vi "Beta 2.1.vi"() -> ()   [LabVIEW 2011]
uses:
  <vilib>/vision/NI_Vision_Development_Module.lvlib
panel:
  in  "OK Button":bool
  in  "Look for":enum16{"Bright Objects", "Dark Objects"}(ring)
  in  "Method":T1(ring)=enum."Inter-class Variance"
  out "Binary":T2(plugin-control)
  out "Threshold Range":cluster{"Lower value":sgl, "Upper value":sgl}={"Lower value"=128.0, "Upper value"=255.0} {"Upper value" format="%.2f"; "Lower value" format="%.2f"}
  in  "Stop":bool
  in  "Browse":bool
  out "XY Graph":cluster{dbl[], dbl[]}(graph)
  out "Original Image":T2(plugin-control)
  out "Path to Image":path
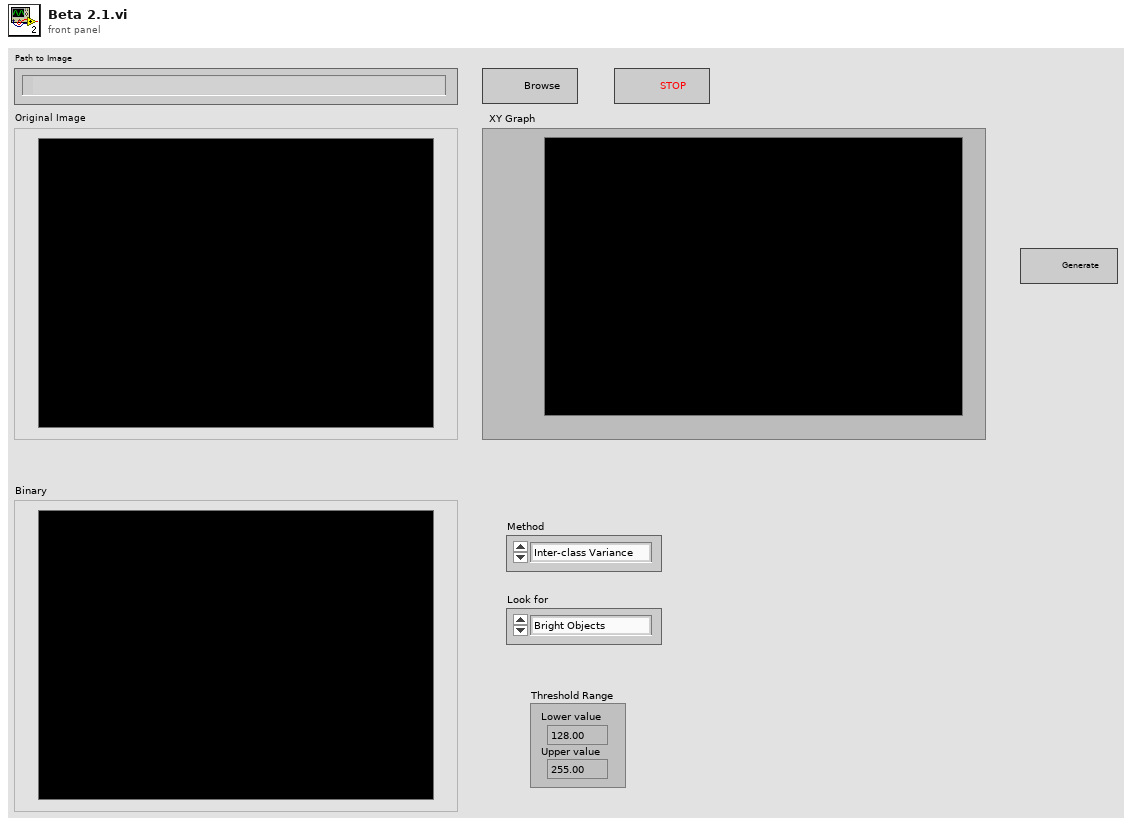
[diagram p1: front panel]
types:
  T1 = enum16{"Clustering", "Entropy", "Metric", "Moments", "Inter-class Variance"}
  T2 = typedef "IMAQ Image.ctl" = refnum<image>
  T3 = typedef "Image Type" = u32
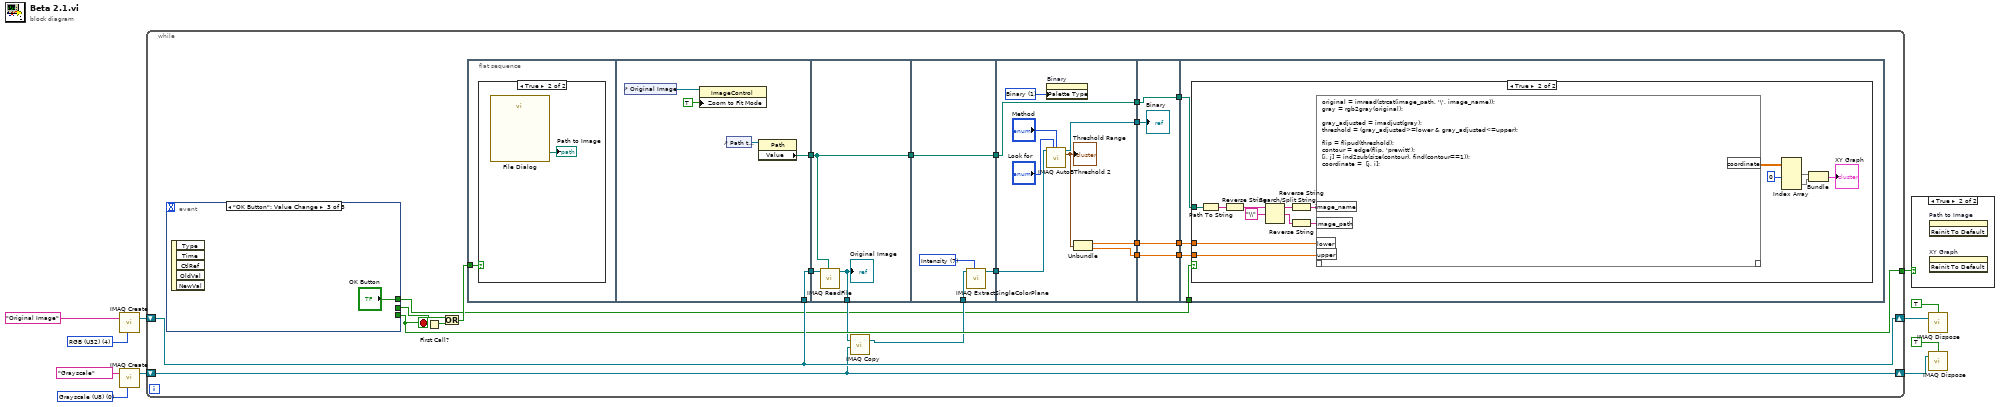
[diagram p0: block diagram]
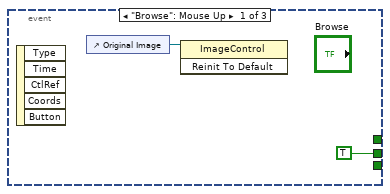
[diagram p3: hidden frame]
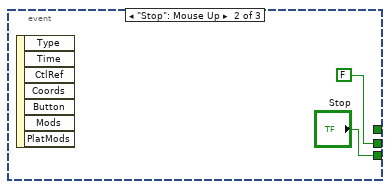
[diagram p4: hidden frame]
diagram:
  w5 = T3 0 items=["Grayscale (U8)", "Grayscale (I16)", "Grayscale (SGL)", "Complex (CSG)", "RGB (U32)", "HSL (U32)", "RGB (U64)", "Grayscale (U16)"] ("Image Type")
  w10 = T3 4 items=["Grayscale (U8)", "Grayscale (I16)", "Grayscale (SGL)", "Complex (CSG)", "RGB (U32)", "HSL (U32)", "RGB (U64)", "Grayscale (U16)"] ("Image Type")
  n1 = call "IMAQ Create"("Image Name"="Original Image", "Image Type"=w10) -> ("New Image"=w9:T2)  [unwired: 3 in, 1 out]
  n2 = call "IMAQ Create"("Image Name"="Grayscale", "Image Type"=w5) -> ("New Image"=w4:T2)  [unwired: 3 in, 1 out]
  n3 = while {
    shift-right: [w27] -> w8
    shift-left: w9 -> [w27]
    tunnel: [w26] -> w7
    shift-right: [w17] -> w2
    shift-left: w4 -> [w17]
    stop <- w26 stop-if-true
    n4 = event shown="[2] \"OK Button\": Value Change" {
      selector: _ -> [_ _ _]
      dyn-events: _ -> [_ _ _]
      timeout: _ -> [_ _ _]
      tunnel: [TRUE FALSE _] -> w31
      tunnel: [_ "Stop" _] -> w26
      tunnel: [_ _ "OK Button"] -> w16
      event "Browse": Mouse Up {
        n5 = event-data() -> ()  [unwired: 1 in, 5 out]
        n6 = control-ref of="Original Image"() -> (w34:refnum<vi>)
        n7 = invoke class="ImageControl" method="Reinit To Default"(reference=w34) -> ()  [unwired: 2 in, 3 out]
      }
      event "Stop": Mouse Up {
        n8 = event-data() -> ()  [unwired: 1 in, 7 out]
      }
      event "OK Button": Value Change {
        n9 = event-data() -> ()  [unwired: 1 in, 5 out]
      }
    }
    n10 = First Call?() -> (First Call?: T/F=w30:bool)
    n11 = Or(x=w31, y=w30) -> (x .or. y?=w29:bool)
    n12 = flat-sequence {
      tunnel: w29 -> [w38]
      tunnel: [w40] -> w32
      tunnel: [w41] -> w28
      tunnel: w27 -> [w40]
      tunnel: w32 -> [w46]
      tunnel: w28 -> [w47]
      tunnel: [w47] -> w25
      tunnel: [w45] -> w19
      tunnel: w25 -> [w51]
      tunnel: [w51] -> w24
      tunnel: [w49] -> w23
      tunnel: w18 -> [w48]
      tunnel: w24 -> [w60]
      tunnel: [w60] -> w22
      tunnel: w23 -> [w59]
      tunnel: [w58] -> w20
      tunnel: [w53] -> w14
      tunnel: [w52] -> w12
      tunnel: w22 -> [w64]
      tunnel: [w64] -> w21
      tunnel: w20 -> [w63]
      tunnel: [w62] -> w15
      tunnel: w14 -> [w62]
      tunnel: [w61] -> w13
      tunnel: w12 -> [w61]
      tunnel: w21 -> [w68]
      tunnel: w16 -> [w67]
      tunnel: w15 -> [w66]
      tunnel: w13 -> [w65]
      frame #0 {
        n13 = case shown="True" w38 {
          frame False {
          }
          frame True {
            n14 = call "File Dialog"() -> ("selected path"=→"Path to Image":path)  [unwired: 12 in, 3 out]
          }
        }
      }
      frame #1 {
        n15 = control-ref of="Original Image"() -> (w44:refnum<vi>)
        n16 = property class="ImageControl"(reference=w44, "Zoom to Fit Mode"=TRUE) -> ()  [unwired: 1 in, 2 out]
        n17 = control-ref of="Path to Image"() -> (w42:refnum<vi>)
        n18 = property class="Path"(reference=w42) -> ("Value"=w41:path)  [unwired: 1 in, 2 out]
      }
      frame #2 {
        n19 = call "IMAQ ReadFile"("File Path"=w47, "Image"=w46) -> ("Image Out"=w45:T2)  [unwired: 5 in, 4 out]
        "Original Image" <- w45
      }
      frame #3 {
        w50 = 7 items=["Red", "Green", "Blue", "Hue", "Saturation", "Luminance", "Value", "Intensity"] ("Color Plane")
        n20 = call "IMAQ ExtractSingleColorPlane"("Color Plane"=w50, "Image Src"=w48) -> ("Image Dst Out"=w49:T2)  [unwired: 8 in, 1 out]
      }
      frame #4 {
        w57 = u32 1 items=["Grayscale", "Binary", "Gradient", "Rainbow", "Temperature", "User Defined"] ("Palette")
        n21 = property on="Binary" class="ImageControl"("Palette Type"=w57) -> ()  [unwired: 2 in, 2 out]
        n22 = call "IMAQ AutoBThreshold 2"("Image Src"=w59, "Look For (Bright Objects)"="Look for", "Method (clustering)"="Method") -> ("Image Dst Out"=w58:T2, "Threshold Range Out"=w54:cluster{"Lower value":sgl, "Upper value":sgl})  [unwired: 10 in, 1 out]
        "Threshold Range" <- w54
        n23 = Unbundle(w54) -> ("Lower value"=w53:sgl, "Upper value"=w52:sgl)
      }
      frame #5 {
        "Binary" <- w63
      }
      frame #6 {
        n24 = case shown="True" w67 {
          tunnel: w68 -> [_ w83]
          tunnel: w66 -> [_ w70]
          tunnel: w65 -> [_ w69]
          frame False {
          }
          frame True {
            n25 = Path To String(path=w83) -> (string=w82:string)
            n26 = Reverse String(1:w82) -> (0:w81:string)
            n27 = Search/Split String(string=w81, search string/char (-)="\\") -> (substring before match=w79:string, match + rest of string=w78:string)  [unwired: 1 in, 1 out]
            n28 = Reverse String(1:w79) -> (0:w77:string)
            n29 = Reverse String(1:w78) -> (0:w76:string)
            n30 = script code="original = imread(strcat(image_path, '\\', image_name));\ngray = rgb2gray(original);\n\ngray_adjusted = imadjust(gray);\nthreshold = (gray_adjusted>=lower & gray_adjusted<=upper);\n\nflip = flipud(threshold);\ncontour = edge(flip, 'prewitt');\n[i, j] = ind2sub(size(contour), find(contour==1));\ncoordinate =  [j, i];"("image_name"=w77, "image_path"=w76, "lower"=w70, "upper"=w69) -> ("coordinate"=w75:dbl[][])  [unwired: 1 in, 1 out]
            n31 = Index Array(array=w75, index (col) #1=0 ("disabled index (col)")) -> (element #1=w74:dbl[], element #2=w73:dbl[])  [unwired: 3 in]
            n32 = Bundle(w74, w73) -> (→"XY Graph":cluster{dbl[], dbl[]})  [unwired: 1 in]
          }
        }
      }
    }
    n33 = call "IMAQ Copy"("Image Dst"=w17, "Image Src"=w19) -> ("Image Dst Out"=w18:T2)  [unwired: 4 in, 1 out]
  }
  n34 = case shown="True" w7 {
    frame False {
    }
    frame True {
      n35 = invoke on="Path to Image" class="Path" method="Reinit To Default"() -> ()  [unwired: 3 in, 3 out]
      n36 = invoke on="XY Graph" class="XYGraph (strict)" method="Reinit To Default"() -> ()  [unwired: 3 in, 3 out]
    }
  }
  n37 = call "IMAQ Dispose"("All Images? (No)"=TRUE, "Image"=w8) -> ()  [unwired: 4 in, 1 out]
  n38 = call "IMAQ Dispose"("All Images? (No)"=TRUE, "Image"=w2) -> ()  [unwired: 4 in, 1 out]
